vi "genererfrekvenssignal0.1.vi"() -> ()   [LabVIEW 2014]
uses:
  <vilib>/MakerHub/LINX/LMH-LINX.lvlib
panel:
  in  "Stop Button":bool
  out "Frequency":dbl(slide) scale=0.0..200.0
  in  "Enable BVM":bool
  in  "Numeric Control":dbl
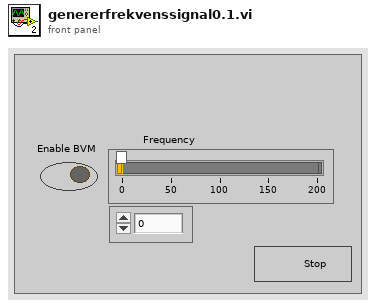
[diagram p1: front panel]
types:
  T1 = typedef "LMH-LINX.lvlib/LINX Ref.ctl" = cluster{"IO":T2, "Interface":T3, "LINX Device Config":T4}
  T2 = typedef "LMH-LINX.lvlib/Platform.ctl" = enum16{"Remote", "Local"}
  T3 = typedef "LMH-LINX.lvlib/Interface.ctl" = enum16{"Serial", "TCP"}
  T4 = typedef "LMH-LINX.lvlib/Device.lvlib/LINX Device Config.ctl" = cluster{"Interface":T3, "COM Port":refnum<visa-resource-name>, "TCP Configuration":T5, "Device Family":u8, "Device ID":u8, "Device Name":string, "TCP Ref":refnum<k5>, "Channels":T6}
  T5 = typedef "LMH-LINX.lvlib/Device.lvlib/TCP Config.ctl" = cluster{"IP Address":string, "Port":u16}
  T6 = typedef "LMH-LINX.lvlib/Channels.ctl" = cluster{"DI":u8[], "DO":u8[], "AI":u8[], "AO":u8[], "PWM":u8[], "QE":u8[], "UART":u8[], "I2C 2":u8[], "SPI":u8[], "CAN":u8[], "Servo":u8[], "AI Ref (V)":dbl, "AI Resolution (Bits)":u8, "AO Ref (V)":dbl, "AO Resolution (Bits)":u8}
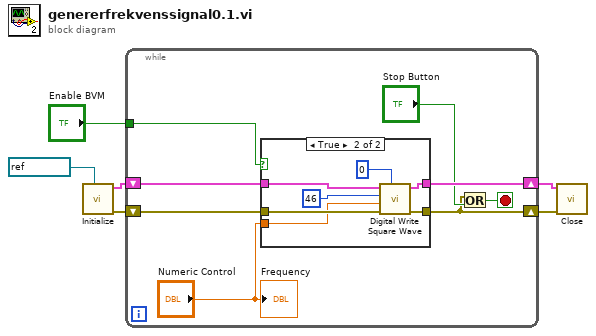
[diagram p0: block diagram]
diagram:
  n1 = call <vilib>:"Initialize.vi"("Serial Port"=refnum<visa-resource-name> "COM5") -> ("Error Out"=w3:errorcluster, "LINX Resource"=w6:T1)  [unwired: 8 in, 1 out]
  n2 = while {
    tunnel: "Enable BVM" -> [w10]
    shift-right: [w13] -> w5
    shift-left: w6 -> [w14]
    shift-right: [w7] -> w4
    shift-left: w3 -> [w12]
    stop <- w9 stop-if-true
    n3 = case shown="True" w10 {
      tunnel: w14 -> [w16 w23]
      tunnel: [w16 w22] -> w13
      tunnel: [w15 w21] -> w7
      tunnel: w12 -> [w15 w20]
      tunnel: "Numeric Control" -> [_ w18]
      frame False {
      }
      frame True {
        n4 = call <vilib>:"Digital Write Square Wave.vi"("Duration (ms)"=u32 0, "Error In"=w20, "Frequency (Hz)"=w18, "Channel"=u8 46, "LINX Resource"=w23) -> ("Error Out"=w21:errorcluster, "LINX Resource"=w22:T1)  [unwired: 5 in]
      }
    }
    n5 = Or(x=w7, y="Stop Button") -> (x .or. y?=w9:bool)
    "Frequency" <- "Numeric Control"
  }
  n6 = call <vilib>:"Close.vi"("Error In"=w4, "LINX Resource"=w5) -> ()  [unwired: 9 in, 1 out]
